vi "Actor Core.vi"(8 "error in":errorcluster, 11 "Nested in":refnum<class "Paquetes.lvclass">) -> (0 "error out":errorcluster, 3 "Actor out":refnum<class "Actor.lvclass">)   [LabVIEW 2020, in "Paquetes.lvlib" / "Paquetes.lvclass"]
doc: "(<B>Filename</B>: Actor Framework.lvlib:Actor.lvclass:Actor Core.vi)\n\nReceives messages to the actor, reacts to them, and initiates any error handling that may shut the actor down.\n\nDescendant classes may override this VI to append parallel tasks for the actor to complete while it handles messages. Overrides use the Call Parent Method node."
uses:
  Paquetes.lvclass
  C:/Program Files (x86)/National Instruments/LabVIEW 2020/vi.lib/ActorFramework/Actor/Actor.lvclass
  <vilib>/ActorFramework/Actor/Actor.lvclass
  <vilib>/ActorFramework/Actor/Actor.lvclass/Actor.ctl
  <vilib>/ActorFramework/Message Enqueuer/Message Enqueuer.lvclass/Message Enqueuer.ctl
  Paquetes.lvclass/Paquetes.ctl
  Paquetes Messages/Servicio seleccionado Msg/Servicio seleccionado Msg.lvclass/Servicio seleccionado Msg.ctl
  <vilib>/ActorFramework/Message Enqueuer/Init from Existing Queue.vi
  <vilib>/ActorFramework/Message Enqueuer/Enqueue.vi
  <vilib>/ActorFramework/Stop Msg/Stop Msg.lvclass
  C:/Program Files (x86)/National Instruments/LabVIEW 2020/vi.lib/ActorFramework/Message/Message.lvclass
  Paquetes Messages/Servicio seleccionado Msg/Servicio seleccionado Msg.lvclass
  <vilib>/ActorFramework/Message Priority Queue/Priority Enqueue.vi
  <vilib>/ActorFramework/Message Enqueuer/Message Enqueuer.lvclass
panel:
  out "String":string
  out "Mensajes":string
  in  "LAVADO TOTAL":bool
  in  "LAVADO DE MOTOR":bool
  in  "ENCERADO":bool
  in  "TAXI":bool
  in  "BASICO":bool
  # "SERVICIOS DISPONIBLES"
  # "MOJADO\n\nENJABONADO\n\nENJUAGE\n\nSECADO\n\nASPIRADO"
  # "MOJADO\n\nENJABONADO\n\nENJUAGE\n\nSECADO\n\nLAVADO \nDE MOTOR"
  # "MOJADO\n\nENJABONADO\n\nENJUAGE\n\nSECADO\n\nASPIRADO\n\nENCERADO"
  # "MOJADO\n\nENJABONADO\n\nENJUAGE\n\nSECADO\n\nASPIRADO\n\nLAVADO DE MOTOR\n\nENCERADO"
  # "MOJADO\n\nENJABONADO\n\nENJUAGE\n\nSECADO"
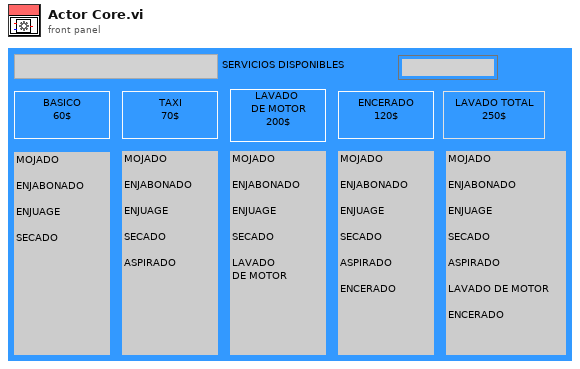
[diagram p1: front panel]
types:
  T1 = cluster{"Stop":refnum<user-event>, "Servicio":refnum<user-event>, "String":refnum<user-event>}
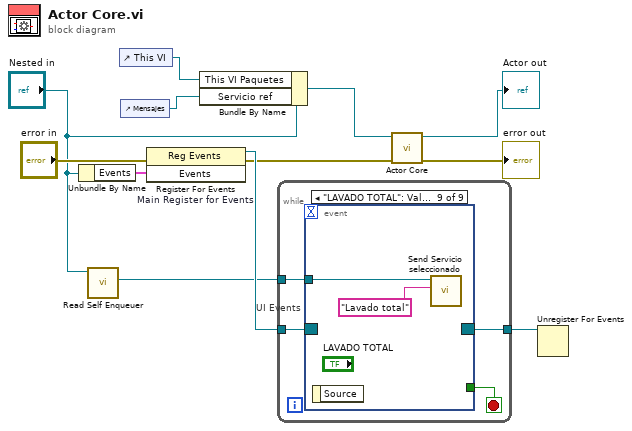
[diagram p0: block diagram]
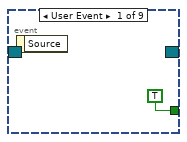
[diagram p2: hidden frame]
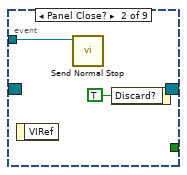
[diagram p3: hidden frame]
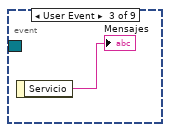
[diagram p4: hidden frame]
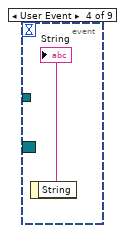
[diagram p5: hidden frame]
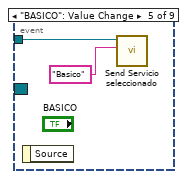
[diagram p6: hidden frame]
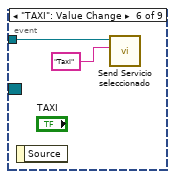
[diagram p7: hidden frame]
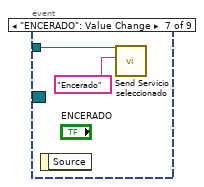
[diagram p8: hidden frame]
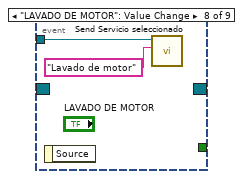
[diagram p9: hidden frame]
diagram:
  n1 = Unbundle By Name("Nested in") -> ("Events"=w9:T1)
  n2 = call <vilib>:"Read Self Enqueuer.vi"("Actor"="Nested in") -> ("Self Enqueuer"=w7:refnum<class "Message Enqueuer.lvclass">)  [unwired: 10 in]
  n3 = control-ref of="This VI"() -> (w1:refnum<vi>)
  n4 = control-ref of="Mensajes"() -> (w2:refnum<vi>)
  n5 = register-events "Main Register for Events"(error in="error in", w9) -> (reference out=w10:refnum<event-registration>, error out=w5:errorcluster)  [unwired: 1 in]
  n6 = Bundle By Name(cluster="Nested in", "This VI Paquetes"=w1, "Servicio ref"=w2) -> (w3:refnum<class "Paquetes.lvclass">)
  n7 = while {
    tunnel: w10 -> [w16]
    tunnel: [w14] -> w8
    tunnel: w7 -> [w13]
    stop <- w15 stop-if-true
    n8 = event "UI Events" shown="[8] \"LAVADO TOTAL\": Value Change" {
      selector: w16 -> [_ _ _ _ _ _ _ _ _]
      dyn-events: [_ _ _ _ _ _ _ _ _] -> w14
      timeout: _ -> [_ _ _ _ _ _ _ _ _]
      tunnel: [TRUE _ _ _ _ _ _ _ _] -> w15
      tunnel: w13 -> [_ w18 _ _ w23 w25 w27 w28 w31]
      event User Event {
        n9 = event-data() -> ()  [unwired: 1 in, 1 out]
      }
      event Panel Close? {
        n10 = event-data() -> ()  [unwired: 1 in, 1 out]
        n11 = call <vilib>:"Send Normal Stop.vi"("Message Enqueuer"=w18) -> ()  [unwired: 10 in, 1 out]
        n12 = event-data("Discard?"=TRUE) -> ()  [unwired: 1 in, 1 out]
      }
      event User Event {
        n13 = event-data() -> ("Servicio"=→"Mensajes":string)  [unwired: 1 in]
      }
      event User Event {
        n14 = event-data() -> ("String"=→"String":string)  [unwired: 1 in]
      }
      event "BASICO": Value Change {
        n15 = event-data() -> ()  [unwired: 1 in, 1 out]
        n16 = call "Send Servicio seleccionado.vi"("Servicio"="Basico", "Message Enqueuer"=w23) -> ()  [unwired: 8 in, 2 out]
      }
      event "TAXI": Value Change {
        n17 = event-data() -> ()  [unwired: 1 in, 1 out]
        n18 = call "Send Servicio seleccionado.vi"("Servicio"="Taxi", "Message Enqueuer"=w25) -> ()  [unwired: 8 in, 2 out]
      }
      event "ENCERADO": Value Change {
        n19 = event-data() -> ()  [unwired: 1 in, 1 out]
        n20 = call "Send Servicio seleccionado.vi"("Servicio"="Encerado", "Message Enqueuer"=w27) -> ()  [unwired: 8 in, 2 out]
      }
      event "LAVADO DE MOTOR": Value Change {
        n21 = event-data() -> ()  [unwired: 1 in, 1 out]
        n22 = call "Send Servicio seleccionado.vi"("Servicio"="Lavado de motor", "Message Enqueuer"=w28) -> ()  [unwired: 8 in, 2 out]
      }
      event "LAVADO TOTAL": Value Change {
        n23 = event-data() -> ()  [unwired: 1 in, 1 out]
        n24 = call "Send Servicio seleccionado.vi"("Servicio"="Lavado total", "Message Enqueuer"=w31) -> ()  [unwired: 8 in, 2 out]
      }
    }
  }
  n25 = call-parent "Actor Core.vi"("error in"=w5, "Actor in"=w3) -> ("error out"=→"error out":errorcluster, "Actor out"=→"Actor out":refnum<class "Actor.lvclass">)  [unwired: 8 in]
  n26 = Unregister For Events(event registration refnum=w8) -> ()  [unwired: 1 in, 1 out]
